vi "Resample Blend.vi"(6 "Length":dbl=1.0, 8 "Speeds":T1={"maxV (fps)"=20.0, "Accel Limit (fps^2)"=20.0, "Initial V (fps)"=0.0, "Sample Period (s)"=0.02, "Jerk Limit (fps^3)"=0.0, "Jerk Distances"={"distance (ft)"=0.0, 0.0, 0.0}, "Jerk Distances"={"distance (ft)"=0.0, 0.0, 0.0}}, 9 "Initial Point":cluster{"x":dbl, "y":dbl, "th":dbl}={"x"=1.0, "y"=2.0, "th"=30.0}, 10 "Point Arrays":cluster{dbl[], dbl[], dbl[]}) -> (0 "Speeds Out":T1={"maxV (fps)"=20.0, "Accel Limit (fps^2)"=20.0, "Initial V (fps)"=0.0, "Sample Period (s)"=0.02, "Jerk Limit (fps^3)"=0.0, "Jerk Distances"={"distance (ft)"=0.0, 0.0, 0.0}, "Jerk Distances"={"distance (ft)"=0.0, 0.0, 0.0}}, 1 "Vel Points":cluster{dbl, dbl}[](array[cluster]), 2 "Points":cluster{dbl, dbl}[](array[cluster]), 3 "Indices":cluster{"Accel Index":i32, "Decel Index":i32})   [LabVIEW 2018]
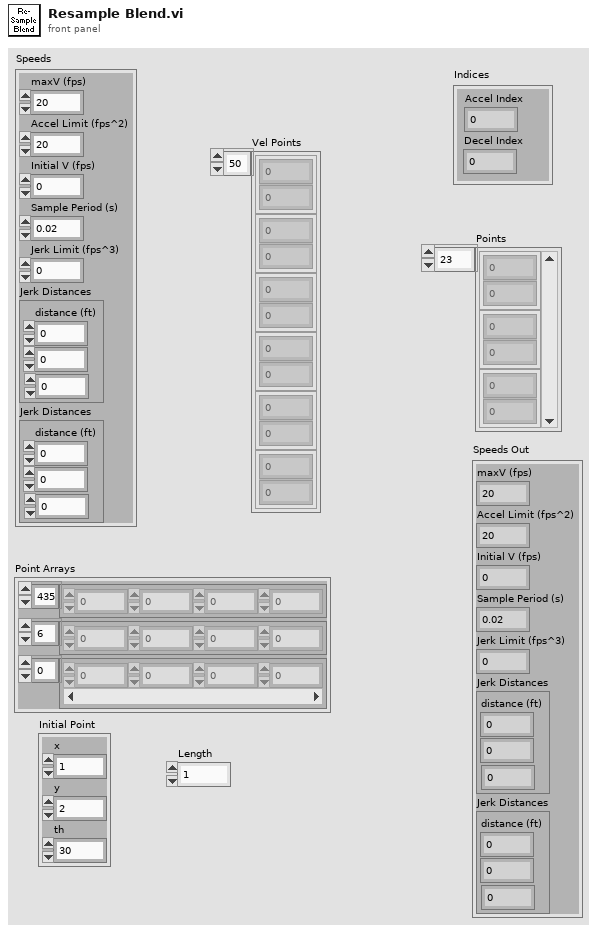
[diagram p1: front panel]
types:
  T1 = cluster{"maxV (fps)":dbl, "Accel Limit (fps^2)":dbl, "Initial V (fps)":dbl, "Sample Period (s)":dbl, "Jerk Limit (fps^3)":dbl, "Jerk Distances":cluster{"distance (ft)":dbl, dbl, dbl}, "Jerk Distances":cluster{"distance (ft)":dbl, dbl, dbl}}
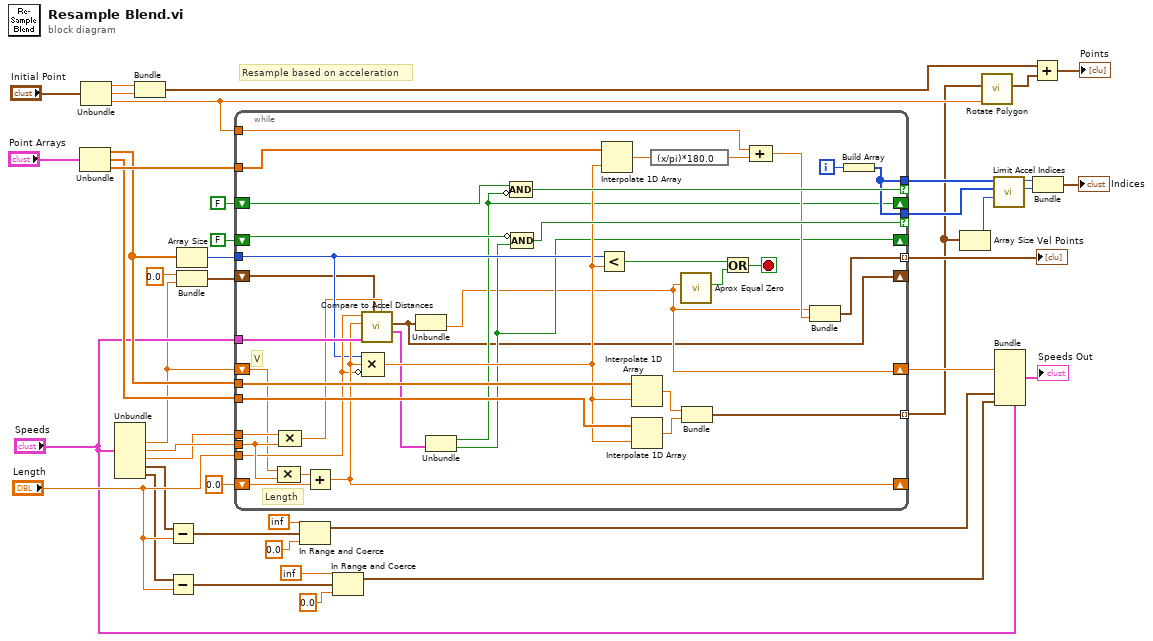
[diagram p0: block diagram]
diagram:
  # "Resample based on acceleration"
  n1 = Unbundle("Point Arrays") -> (w36:dbl[], w37:dbl[], w38:dbl[])
  n2 = Unbundle("Initial Point") -> ("x"=w33:dbl, "y"=w34:dbl, "th"=w32:dbl)
  n3 = Unbundle("Speeds") -> ("Initial V (fps)"=w1:dbl, "Sample Period (s)"=w42:dbl, "Jerk Limit (fps^3)"=w4:dbl, "Jerk Distances"=w8:cluster{"distance (ft)":dbl, dbl, dbl}, "Jerk Distances"=w9:cluster{"distance (ft)":dbl, dbl, dbl})  [unwired: 2 out]
  n4 = Bundle("x"=w33, "y"=w34) -> (w31:cluster{"x":dbl, "y":dbl})  [unwired: 1 in]
  n5 = Subtract(x=w8, y="Length") -> (x-y=w28:cluster{"distance (ft)":dbl, dbl, dbl})
  n6 = Subtract(x=w9, y="Length") -> (x-y=w24:cluster{"distance (ft)":dbl, dbl, dbl})
  n7 = Array Size(array=w36) -> (size(s)=w22:i32)
  n8 = Bundle(0.0, "Initial V (fps)"=w1) -> (w3:cluster{dbl, "Initial V (fps)":dbl})  [unwired: 1 in]
  n9 = while {
    tunnel: w36 -> [w79]
    tunnel: w37 -> [w78]
    tunnel: [w75] -> w15 mode=indexing
    tunnel: w42 -> [w59]
    shift-right: [w45] -> w41
    shift-left: w1 -> [w47]
    tunnel: w4 -> [w74]
    tunnel: w22 -> [w52]
    tunnel: w38 -> [w73]
    tunnel: w32 -> [w71]
    shift-right: [w49] -> _
    shift-left: FALSE -> [w69]
    tunnel: [w56] -> w19 if=w68
    tunnel: "Length" -> [w54]
    tunnel: "Speeds" -> [w67]
    shift-right: [w48] -> _
    shift-left: FALSE -> [w66]
    tunnel: [w56] -> w18 if=w65
    tunnel: [w62] -> w20 mode=indexing
    shift-right: [w55] -> _
    shift-left: 0.0 -> [w60]
    shift-right: [w44] -> _
    shift-left: w3 -> [w43]
    i -> [w57]
    stop <- w63 stop-if-true
    # "Length"
    # "V"
    n10 = Compound Arithmetic op=MULTIPLY(w47, w59) -> (w58:dbl)
    n11 = Compound Arithmetic op=MULTIPLY(w74, w59) -> (w46:dbl)
    n12 = Add(x=w58, y=w60) -> (x+y=w55:dbl)
    n13 = call "Compare to Accel Distances.vi"("dA"=w46, "Values"=w43, "Speeds"=w67, "Current  Length"=w55, "Total Segment Length"=w54) -> ("Ends"=w50:cluster{"Accel End":bool, "Decel End":bool}, "Values out"=w44:cluster{"accel":dbl, "velocity":dbl})  [unwired: 3 in, 2 out]
    n14 = Compound Arithmetic op=MULTIPLY(w52, w55, invert w54) -> (w53:dbl)
    n15 = Unbundle(w44) -> ("velocity"=w45:dbl)  [unwired: 1 out]
    n16 = Unbundle(w50) -> ("Accel End"=w49:bool, "Decel End"=w48:bool)
    n17 = Compound Arithmetic op=AND(w69, invert w49) -> (w68:bool)
    n18 = Compound Arithmetic op=AND(invert w66, w48) -> (w65:bool)
    n19 = Less?(x=w52, y=w53) -> (x < y?=w64:bool)
    n20 = Interpolate 1D Array(1:w53, 2:w73) -> (0:w72:dbl)
    n21 = Interpolate 1D Array(1:w53, 2:w79) -> (0:w77:dbl)
    n22 = Interpolate 1D Array(1:w53, 2:w78) -> (0:w76:dbl)
    n23 = expression code="(x/pi)*180.0" ("radians to degrees")(w72) -> (w70:dbl)
    n24 = call "Aprox Equal Zero.vi"("maxV (fps)"=w45) -> ("Boolean"=w51:bool)  [unwired: 10 in]
    n25 = Bundle(w77, w76) -> (w75:cluster{dbl, dbl})  [unwired: 1 in]
    n26 = Or(x=w64, y=w51) -> (x .or. y?=w63:bool)
    n27 = Compound Arithmetic op=ADD(w71, w70) -> (w61:dbl)
    n28 = Bundle("velocity"=w45, w61) -> (w62:cluster{"velocity":dbl, dbl})  [unwired: 1 in]
    n29 = Build Array(w57) -> (w56:i32[])
  }
  "Vel Points" <- w20
  n30 = In Range and Coerce(upper limit=inf, x=w28, lower limit=0.0) -> (coerced(x)=w6:cluster{"distance (ft)":dbl, dbl, dbl})  [unwired: 1 out]
  n31 = In Range and Coerce(upper limit=inf, x=w24, lower limit=0.0) -> (coerced(x)=w7:cluster{"distance (ft)":dbl, dbl, dbl})  [unwired: 1 out]
  n32 = Array Size(array=w15) -> (size(s)=w14:i32)
  n33 = call "Rotate Polygon.vi"("Angle"=w32, "polygon 2"=w15) -> ("polygon"=w30:cluster{dbl, dbl}[])  [unwired: 9 in]
  n34 = call "Limit Accel Indices.vi"("Size"=w14, "Decel"=w18, "Accel"=w19) -> ("Decel Index"=w16:i32, "Accel Index"=w17:i32)  [unwired: 7 in]
  n35 = Bundle(cluster="Speeds", "Initial V (fps)"=w41, "Jerk Distances"=w6, "Jerk Distances"=w7) -> (→"Speeds Out":T1)  [unwired: 4 in]
  n36 = Add(x=w31, y=w30) -> (x+y=→"Points":cluster{dbl, dbl}[])
  n37 = Bundle("Accel Index"=w17, "Decel Index"=w16) -> (→"Indices":cluster{"Accel Index":i32, "Decel Index":i32})  [unwired: 1 in]
